vi "calculator.vi"() -> ()   [LabVIEW 2016]
uses:
  <vilib>/Instr/_visa.llb/VISA Configure Serial Port (Instr).vi
panel:
  in  "write buffer":string
  out "read buffer 2":string
  out "error out 2":errorcluster
  out "VISA resource name out 2":refnum<visa-resource-name>
  in  "flow control (0:none)":u16(ring) items=["None", "XON/XOFF", "RTS/CTS", "XON/XOFF & RTS/CTS", "DTR/DSR", "XON/XOFF & DTR/DSR"]
  in  "stop bits (10: 1 bit)":u16(ring)=10 items=["1.0"=10, "1.5"=15, "2.0"=20]
  in  "error in (no error) 2":errorcluster
  in  "parity (0:none)":enum16{"None", "Odd", "Even", "Mark", "Space"}(ring)
  in  "data bits (8)":u16=8 min=5 max=8 step=1
  in  "baud rate (9600)":u32=9600
  in  "Enable Termination\nChar (T)":bool=TRUE
  in  "termination char\n(0xA = '\\n' = LF)":u8=10 format="%.0x"
  in  "timeout (10sec)":u32=10000
  in  "VISA resource name 2":refnum<visa-resource-name>
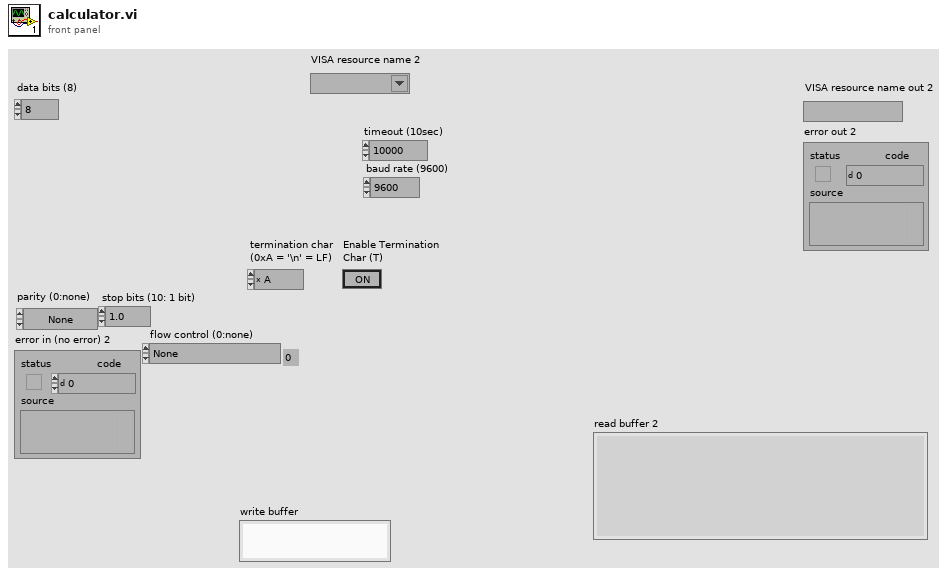
[diagram p1: front panel]
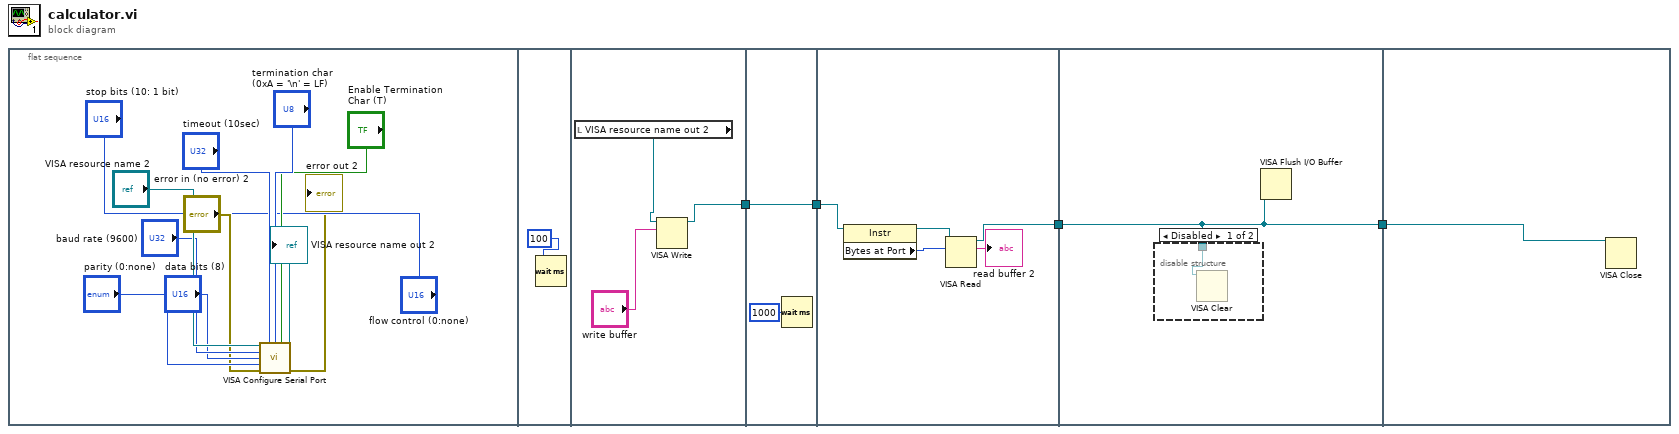
[diagram p0: block diagram]
diagram:
  n1 = flat-sequence {
    tunnel: [w19] -> w4
    tunnel: w4 -> [w22]
    tunnel: [w22] -> w3
    tunnel: w3 -> [w27]
    tunnel: [w23] -> w2
    tunnel: w2 -> [w28]
    tunnel: [w28] -> w1
    tunnel: w1 -> [w30]
    frame #0 {
      n2 = call-poly "VISA Configure Serial Port"("VISA resource name"="VISA resource name 2", "timeout (10sec)"="timeout (10sec)", "termination char\n(0xA = '\\n' = LF)"="termination char\n(0xA = '\\n' = LF)", "Enable Termination\nChar (T)"="Enable Termination\nChar (T)", "baud rate (9600)"="baud rate (9600)", "data bits (8)"="data bits (8)", "parity (0:none)"="parity (0:none)", "error in (no error)"="error in (no error) 2", "stop bits (10: 1 bit)"="stop bits (10: 1 bit)", "flow control (0:none)"="flow control (0:none)") -> ("VISA resource name out"=→"VISA resource name out 2":refnum<visa-resource-name>, "error out"=→"error out 2":errorcluster)  [unwired: 4 in]
    }
    frame #1 {
      n3 = Wait (ms)(milliseconds to wait=u32 100) -> ()  [unwired: 1 out]
    }
    frame #2 {
      n4 = local read "VISA resource name out 2"() -> (w20:refnum<visa-resource-name>)
      n5 = VISA Write(VISA resource name=w20, write buffer="write buffer") -> (VISA resource name out=w19:refnum<visa-resource-name>)  [unwired: 1 in, 2 out]
    }
    frame #3 {
      n6 = Wait (ms)(milliseconds to wait=u32 1000) -> ()  [unwired: 1 out]
    }
    frame #4 {
      n7 = property class="Instr"(reference=w27) -> (reference out=w26:refnum<visa-resource-name>, "Bytes at Port"=w25:u32)  [unwired: 1 in, 1 out]
      n8 = VISA Read(VISA resource name=w26, byte count=w25) -> (VISA resource name out=w23:refnum<visa-resource-name>, read buffer=→"read buffer 2":string)  [unwired: 1 in, 2 out]
    }
    frame #5 {
      n9 = disable-structure shown="Disabled" {
        disable-tunnel: w28 -> [w29 _]
        frame Disabled {
          n10 = VISA Clear(VISA resource name=w29) -> ()  [unwired: 1 in, 2 out]
        }
        frame Enabled {
        }
      }
      n11 = VISA Flush I/O Buffer(VISA resource name=w28) -> ()  [unwired: 2 in, 2 out]
    }
    frame #6 {
      n12 = VISA Close(VISA resource name=w30) -> ()  [unwired: 1 in, 1 out]
    }
  }
